vi "Array of Device Info to Channel Data.vi"(1 "Array of Devices":T1[](array[typedef])) -> (0 "Device Channels":i32[](array[numeric]))   [LabVIEW 2014, in "SPI Engine Scripting.lvlib"]
doc: "Creates an array where each element corresponds to a device on bus currently being scripted and the value in each element corresponds to the number of channels on that device."
uses:
  SPI Engine Scripting.lvlib
  Controls/Device Information.ctl
  <vilib>/LabVIEW Icon API/API_Text.ctl
  <vilib>/LabVIEW Icon API/LabVIEW Icon API.lvlib
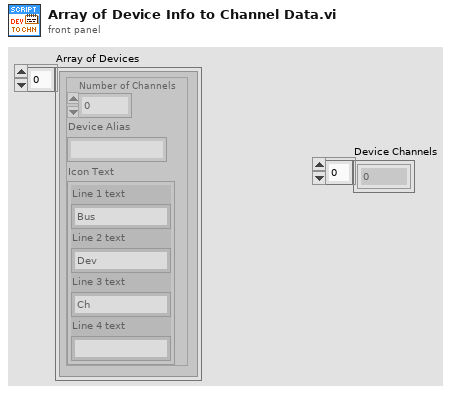
[diagram p1: front panel]
types:
  T1 = typedef "Device Information.ctl" = cluster{"Number of Channels":i32, "Device Alias":string, "Icon Text":T2}
  T2 = typedef "LabVIEW Icon API.lvlib/API_Text.ctl" = cluster{"Line 1 text":string, "Line 2 text":string, "Line 3 text":string, "Line 4 text":string}
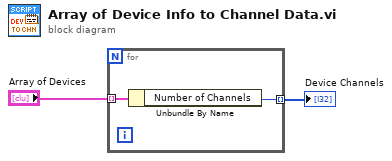
[diagram p0: block diagram]
diagram:
  n1 = for {
    tunnel: "Array of Devices" -> [w4] mode=indexing
    tunnel: [w3] -> w2 mode=indexing
    n2 = Unbundle By Name(w4) -> ("Number of Channels"=w3:i32)
  }
  "Device Channels" <- w2
